vi "nii_file_read_dim.vi"(8 "error in (no error)":errorcluster, 11 "file (use dialog)":path) -> (0 "error out":errorcluster, 1 "variant":variant, 2 "Data":T1 {"slice orientation" items=["transverse unflipped", "coronal unflipped", "sagittal unflipped", "transverse flipped", "coronal flipped", "sagittal flipped"]})   [LabVIEW 2014]
uses:
  nii_read.vi
  control/head_data.ctl
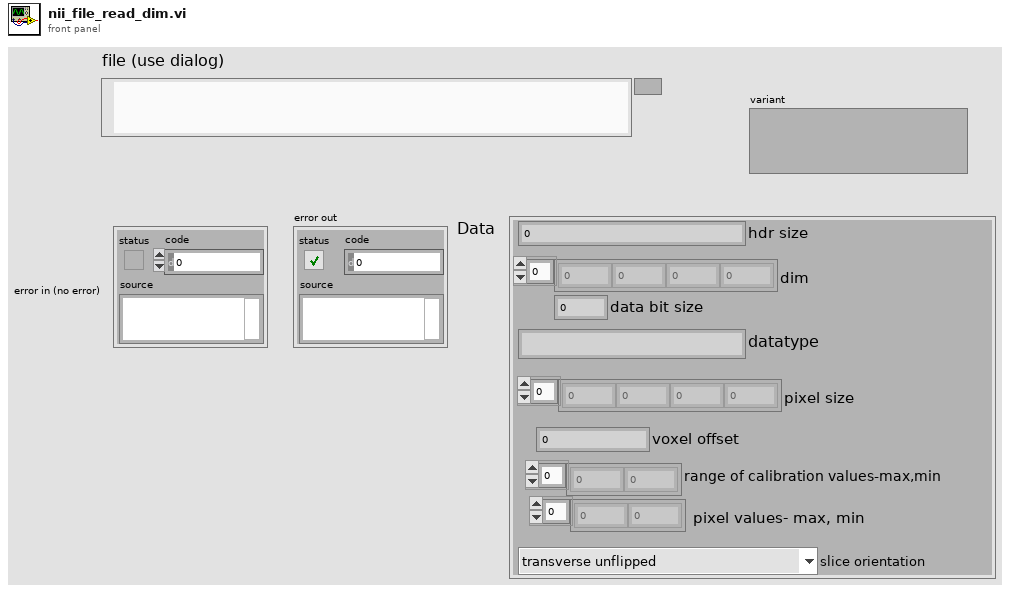
[diagram p1: front panel]
types:
  T1 = typedef "head_data.ctl" = cluster{"hdr size":i32, "dim":i32[], "data bit size":i32, "datatype":string, "pixel size ":sgl[], "voxel offset":sgl, "range of calibration values-max,min":sgl[], " pixel values- max, min":sgl[], "slice orientation":u16}
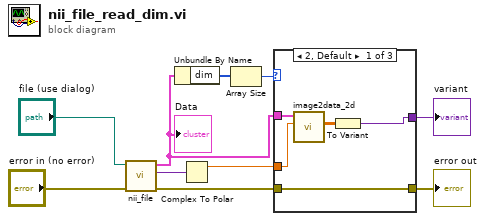
[diagram p0: block diagram]
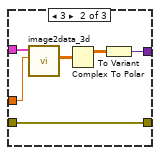
[diagram p2: hidden frame]
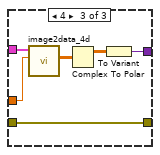
[diagram p3: hidden frame]
diagram:
  n1 = call-poly "nii_file.vi"("error in (no error)"="error in (no error)", "file (use dialog)"="file (use dialog)") -> ("error out"=w5:errorcluster, "variant"=w2:variant, "Data"=w10:T1)  [unwired: 5 in, 2 out]
  "Data" <- w10
  n2 = Unbundle By Name(w10) -> ("dim"=w9:i32[])
  n3 = Complex To Polar(r * e^(i*theta)=w2) -> (r=w1:dbl)  [unwired: 1 out]
  n4 = Array Size(array=w9) -> (size(s)=w8:i32)
  n5 = case shown="2, Default" w8 {
    tunnel: [w15 w20 w26] -> w3
    tunnel: w10 -> [w13 w21 w27]
    tunnel: w5 -> [w14 w19 w25]
    tunnel: [w14 w19 w25] -> w4
    tunnel: w1 -> [w12 w16 w22]
    frame 2, Default {
      n6 = call "image2data_2d.vi"("image_1d"=w12, "Data"=w13) -> ("image_2d"=w11:dbl[][])  [unwired: 8 in, 1 out]
      n7 = To Variant(anything=w11) -> (Variant=w15:variant)
    }
    frame 3 {
      n8 = call "image2data_3d.vi"("image_1d"=w16, "Data"=w21) -> ("Array"=w17:dbl[][][])  [unwired: 8 in, 1 out]
      n9 = Complex To Polar(r * e^(i*theta)=w17) -> (r=w18:dbl[][][])  [unwired: 1 out]
      n10 = To Variant(anything=w18) -> (Variant=w20:variant)
    }
    frame 4 {
      n11 = call "image2data_4d.vi"("image_1d"=w22, "Data"=w27) -> ("Array"=w23:dbl[][][][])  [unwired: 8 in, 1 out]
      n12 = Complex To Polar(r * e^(i*theta)=w23) -> (r=w24:dbl[][][][])  [unwired: 1 out]
      n13 = To Variant(anything=w24) -> (Variant=w26:variant)
    }
  }
  "error out" <- w4
  "variant" <- w3
